vi "Set Columns.vi"(3 "error in (no error)":errorcluster, 4 "Columns in":refnum<class "Column.lvclass">[](array[class]), 5 "Pulseblaster in":refnum<class "Slave_Pulseblaster.lvclass">) -> (0 "error out":errorcluster, 1 "Pulseblaster out":refnum<class "Slave_Pulseblaster.lvclass">)   [LabVIEW 2013, in "Slave_Pulseblaster.lvclass"]
uses:
  Slave_Pulseblaster.lvclass
  ColumnVIs/Column/Column.lvclass
  <vilib>/Utility/error.llb/DialogType.ctl
  Device/Device.lvclass
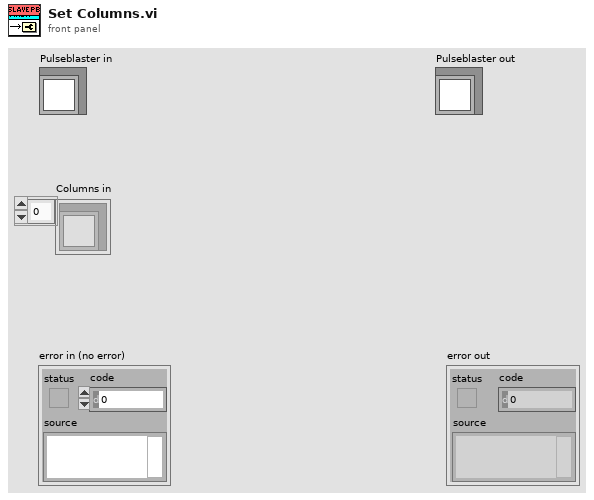
[diagram p1: front panel]
types:
  T1 = typedef "DialogType.ctl" = u16
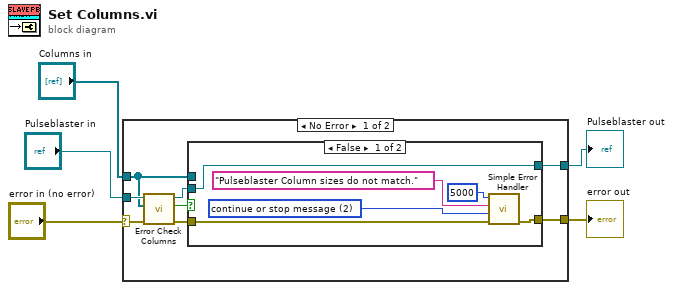
[diagram p0: block diagram]
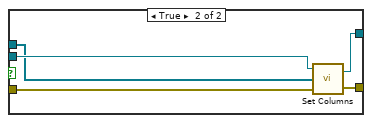
[diagram p2: hidden frame]
diagram:
  n1 = case shown="No Error" "error in (no error)" {
    selector: "error in (no error)" -> [w11 w25]
    tunnel: [w13 w25] -> w2
    tunnel: [w12 w26] -> w1
    tunnel: "Columns in" -> [w7 _]
    tunnel: "Pulseblaster in" -> [w9 w26]
    frame No Error {
      n2 = call-dynamic "Error Check Columns.vi"("error in (no error)"=w11, "Columns in"=w7, "Slave_Pulseblaster in"=w9) -> ("error out"=w10:errorcluster, "Columns OK"=w6:bool, "Slave_Pulseblaster out"=w8:refnum<class "Slave_Pulseblaster.lvclass">)  [unwired: 6 in]
      n3 = case shown="False" w6 {
        tunnel: [w15 w20] -> w13
        tunnel: [w17 w21] -> w12
        tunnel: w7 -> [_ w23]
        tunnel: w8 -> [w17 w24]
        tunnel: w10 -> [w16 w22]
        frame False {
          w18 = T1 2 items=["no dialog", "OK message", "continue or stop message", "OK message + warnings", "continue/stop + warnings"] ("type of dialog (OK msg:1)")
          n4 = call <vilib>:"Simple Error Handler.vi"("error code (no error:0)"=5000, "error source (\" \")"="Pulseblaster Column sizes do not match." ("message"), "type of dialog (OK msg:1)"=w18, "error in (no error)"=w16) -> ("error out"=w15:errorcluster)  [unwired: 1 in, 4 out]
        }
        frame True {
          n5 = call-parent "Set Columns.vi"("error in (no error)"=w22, "Columns"=w23, "Device in"=w24) -> ("error out"=w20:errorcluster, "Device out"=w21:refnum<class "Slave_Pulseblaster.lvclass">)  [unwired: 1 in]
        }
      }
    }
    frame Error {
    }
  }
  "error out" <- w2
  "Pulseblaster out" <- w1
